vi "Position_to_Velocity.vi"(0 "Position":dbl, 1 "d":dbl, 2 "LoopTime":dbl) -> (7 "Velocity":dbl)   [LabVIEW 2019]
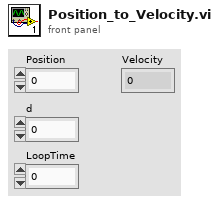
[diagram p1: front panel]
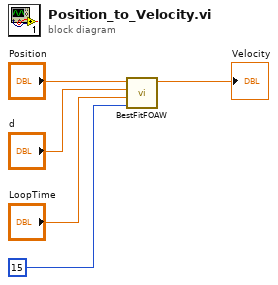
[diagram p0: block diagram]
diagram:
  n1 = call "BestFitFOAW.vi"("y_k"="Position", "d"="d", "T"="LoopTime", "n_max"=15) -> ("vel estimation"=→"Velocity":dbl)  [unwired: 5 in, 1 out]
